vi "重排数组.vi"(8 "新索引顺序":i32[](array[numeric]), 11 "原数组":variant[](array[variant])) -> (3 "排序后数组":variant[](array[variant]))   [LabVIEW 2017]
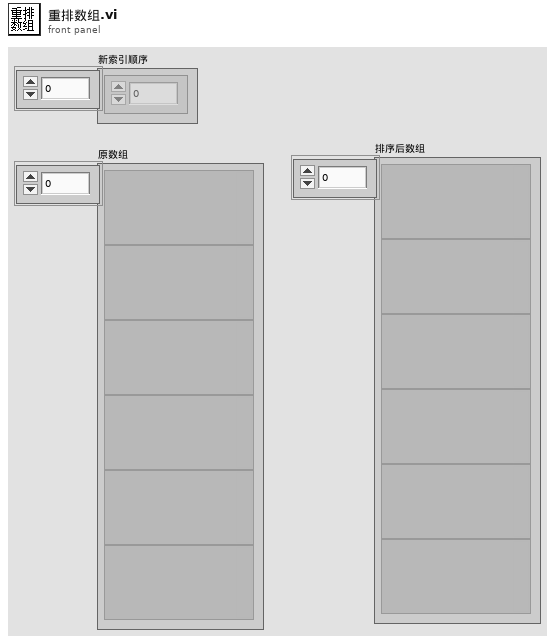
[diagram p1: front panel]
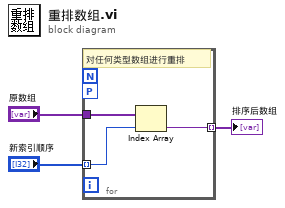
[diagram p0: block diagram]
diagram:
  n1 = for {
    tunnel: "原数组" -> [w6]
    tunnel: "新索引顺序" -> [w5] mode=indexing
    tunnel: [w4] -> w1 mode=indexing
    workers-P: _ -> [_]
    # "对任何类型数组进行重排"
    n2 = Index Array(array=w6, index=w5) -> (element=w4:variant)
  }
  "排序后数组" <- w1
